vi "Read Formatted JSON.vi"(6 "Pretty Print Levels (5)":i32=5, 8 "error in (no error)":errorcluster, 11 "CycloneDX SBOM in":refnum<class "CycloneDX JSON.lvclass">) -> (0 "error out":errorcluster, 2 "JSON":string, 3 "CycloneDX SBOM out":refnum<class "CycloneDX JSON.lvclass">)   [LabVIEW 2017, in "LabVIEW CycloneDX SBOM.lvlib" / "CycloneDX JSON.lvclass"]
doc: "Read the JSON representation as pretty-printed JSON."
uses:
  CycloneDX JSON.lvclass
  CycloneDX JSON.lvclass/CycloneDX JSON.ctl
  <vilib>/JDP Science/JSONtext/JSONtext.lvlib
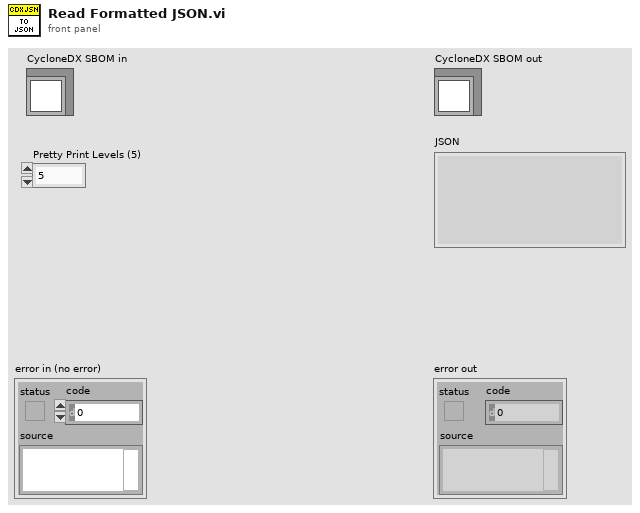
[diagram p1: front panel]
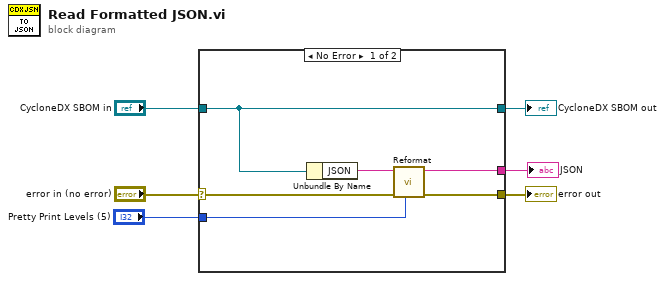
[diagram p0: block diagram]
diagram:
  n1 = case shown="No Error" "error in (no error)" {
    selector: "error in (no error)" -> [w10 w14]
    tunnel: [w9 w14] -> w5
    tunnel: [w12 w13] -> w3
    tunnel: "CycloneDX SBOM in" -> [w12 w13]
    tunnel: [w8 _] -> w2
    tunnel: "Pretty Print Levels (5)" -> [w7 _]
    frame No Error {
      n2 = Unbundle By Name(w12) -> ("JSON"=w11:string)
      n3 = call <vilib>:"Reformat.vi"("Pretty Print Levels"=w7, "error in (no error)"=w10, "JSON"=w11) -> ("error out"=w9:errorcluster, "<JSON>First JSON Value\n\n<JSON>"=w8:string)  [unwired: 5 in, 2 out]
    }
    frame Error {
    }
  }
  "error out" <- w5
  "CycloneDX SBOM out" <- w3
  "JSON" <- w2
